vi "Get Data I16.vi"(8 "error in (no error)":errorcluster, 11 "Ni-Scope Digitizer in":refnum<class "Ni-Scope Digitizer.lvclass">) -> (0 "error out":errorcluster, 1 "Current read position":i32, 2 "Data out":i16[][](array[numeric]), 3 "Ni-Scope Digitizer out":refnum<class "Ni-Scope Digitizer.lvclass">, 4 "Finished":bool)   [LabVIEW 2015, in "Ni-Scope Digitizer.lvclass"]
uses:
  Ni-Scope Digitizer.lvclass
  Instruments/Pulse Driver/Pulse Driver.lvclass/Pulse Driver.ctl
  Ni-Scope Digitizer.lvclass/Ni-Scope Digitizer.ctl
  Instruments/Pulse Driver/Write t0.vi
  Instruments/Pulse Driver/Write dt.vi
  Instruments/Pulse Driver/Write Scaling coefficients.vi
  Instruments/Pulse Driver/Read Samples per channel.vi
  Instruments/Pulse Driver/Read User Configuration.vi
  Instruments/Pulse Driver/Read Current read position.vi
  Instruments/Pulse Driver/Read Samples per read.vi
  <instrlib>/niScope/Acquire/Fetch/niScope Multi Fetch Binary 16.vi
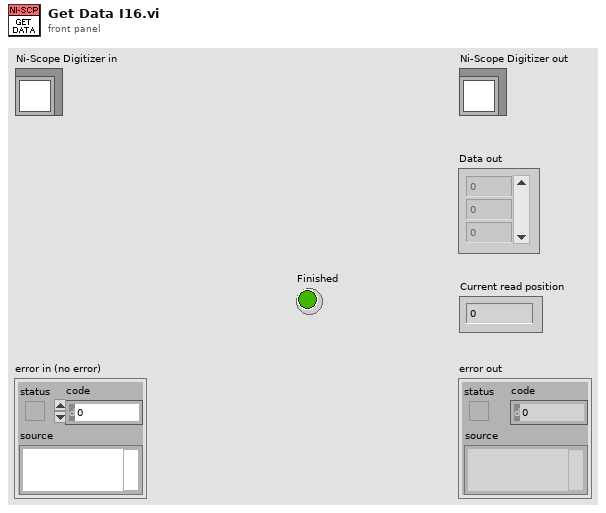
[diagram p1: front panel]
types:
  T1 = typedef "Pusle Driver Configuration.ctl" = cluster{"Pre-trigger duration":dbl, "Post-trigger duration":dbl, "Rate":dbl, "Ranges":dbl[], "Re-name channels":string[], "Active channels":string, "External clock":bool}
  T2 = cluster{"actualSamples":i32, "absoluteInitialX":dbl, "relativeInitialX":dbl, "xIncrement":dbl, "offset":dbl, "gain":dbl, "reserved1":dbl, "reserved2":dbl}[]
  T3 = cluster{"actualSamples":i32, "absoluteInitialX":dbl, "relativeInitialX":dbl, "xIncrement":dbl, "offset":dbl, "gain":dbl, "reserved1":dbl, "reserved2":dbl}
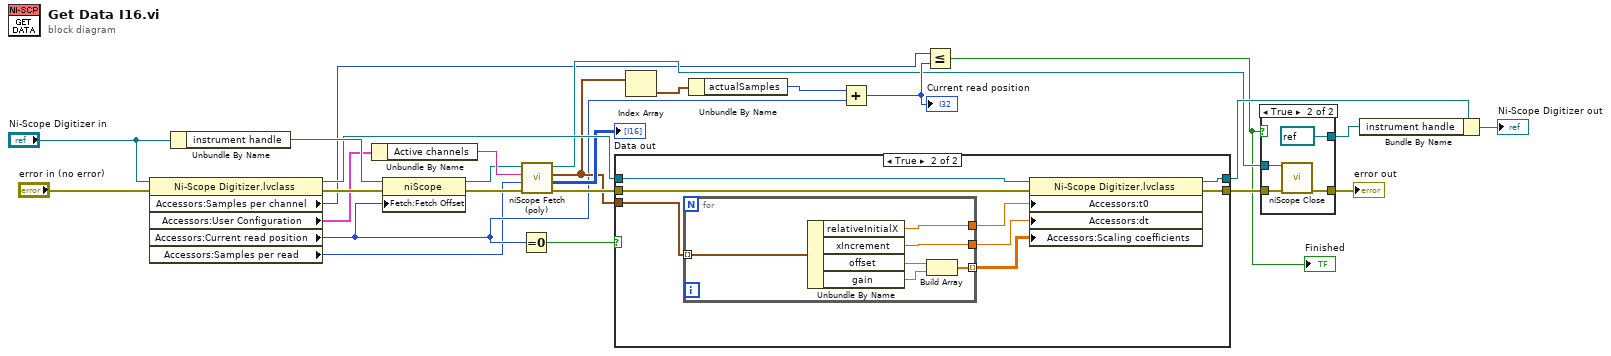
[diagram p0: block diagram]
diagram:
  n1 = property class="Ni-Scope Digitizer.lvclass"(reference="Ni-Scope Digitizer in", error in="error in (no error)") -> (reference out=w18:refnum<class "Ni-Scope Digitizer.lvclass">, error out=w21:errorcluster, "Accessors:Samples per channel"=w4:i32, "Accessors:User Configuration"=w3:T1, "Accessors:Current read position"=w5:i32, "Accessors:Samples per read"=w2:i32)
  n2 = Unbundle By Name("Ni-Scope Digitizer in") -> ("instrument handle"=w24:refnum<k15>)
  n3 = Unbundle By Name(w3) -> ("Active channels"=w26:string)
  n4 = property class="niScope"(reference=w24, error in=w21, "Fetch:Fetch Offset"=w5) -> (reference out=w23:refnum<k15>, error out=w22:errorcluster)
  n5 = Equal To 0?(x=w5) -> (x = 0?=w19:bool)
  n6 = call-poly <instrlib>:"niScope Fetch (poly).vi"("error in"=w22, "numSamples"=w2, "channels"=w26, "instrument handle"=w23) -> ("error out"=w17:errorcluster, "wfm"=→"Data out":i16[][], "wfm info"=w14:T2, "instrument handle out"=w10:refnum<k15>)  [unwired: 4 in]
  n7 = case shown="True" w19 {
    tunnel: w14 -> [_ w36]
    tunnel: w18 -> [w28 w35]
    tunnel: w17 -> [w27 w34]
    tunnel: [w28 w30] -> w16
    tunnel: [w27 w29] -> w9
    frame False {
    }
    frame True {
      n8 = for {
        tunnel: w36 -> [w42] mode=indexing
        tunnel: [w41] -> w33
        tunnel: [w40] -> w32
        tunnel: [w37] -> w31 mode=indexing
        n9 = Unbundle By Name(w42) -> ("relativeInitialX"=w41:dbl, "xIncrement"=w40:dbl, "offset"=w39:dbl, "gain"=w38:dbl)
        n10 = Build Array(w39, w38) -> (w37:dbl[])
      }
      n11 = property class="Ni-Scope Digitizer.lvclass"(reference=w35, error in=w34, "Accessors:t0"=w33, "Accessors:dt"=w32, "Accessors:Scaling coefficients"=w31) -> (reference out=w30:refnum<class "Ni-Scope Digitizer.lvclass">, error out=w29:errorcluster)
    }
  }
  n12 = Index Array(array=w14) -> (element=w13:T3)  [unwired: 1 in]
  n13 = Unbundle By Name(w13) -> ("actualSamples"=w12:i32)
  n14 = Add(x=w12, y=w5) -> (x+y=w11:i32)
  "Current read position" <- w11
  n15 = Less Or Equal?(x=w4, y=w11) -> (x <= y?=w1:bool)
  "Finished" <- w1
  n16 = case shown="True" w1 {
    tunnel: [w44 w48] -> w8
    tunnel: w10 -> [w43 w47]
    tunnel: w9 -> [w44 w46]
    tunnel: [w43 refnum<k15> refnum ("instrument handle out")] -> w6
    frame False {
    }
    frame True {
      n17 = call <instrlib>:"niScope Close.vi"("instrument handle"=w47, "error in"=w46) -> ("error out"=w48:errorcluster)  [unwired: 13 out]
    }
  }
  "error out" <- w8
  n18 = Bundle By Name(cluster=w16, "instrument handle"=w6) -> (→"Ni-Scope Digitizer out":refnum<class "Ni-Scope Digitizer.lvclass">)
